vi "Counter_PulseWidthMeasurement.vi"() -> ()   [LabVIEW 2020]
uses:
  <userlib>/DAQNavi Polymorphic VI/create/DAQNavi Create Channel(CI-PulseWidth).vi
  <userlib>/DAQNavi Polymorphic VI/read/DAQNavi Read (Counter Pulse Width 1Chan 1Samp).vi
panel:
  in  "physical channels":string="PCI-1780,BID#0/cntr0" caption="property value"
  out "data":cluster{"high period":dbl, "low period":dbl}
  in  "stop":bool
  # "Please modify physical channels in Channel Parameters through DAQNavi Property Assistant VI  in block diagram."
  # "Channel Parameters"
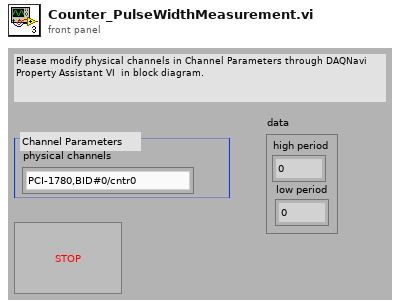
[diagram p1: front panel]
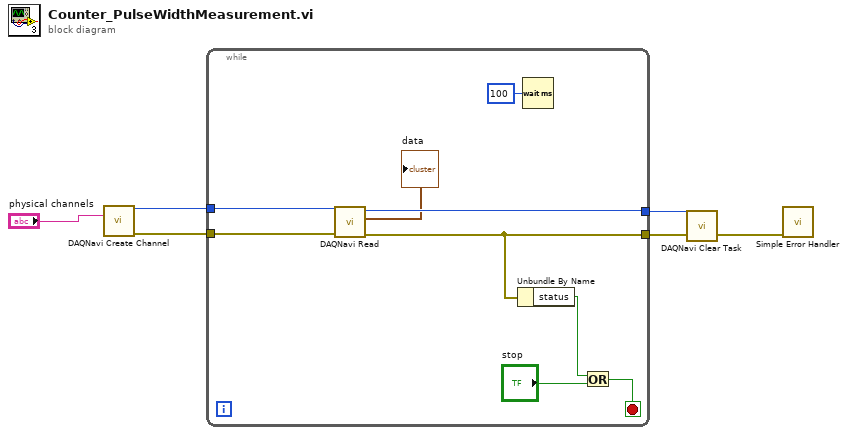
[diagram p0: block diagram]
diagram:
  n1 = call-poly <userlib>:"DAQNavi Create Channel.vi"("physical channels"="physical channels") -> ("task out"=w5:i32, "error out"=w4:errorcluster)  [unwired: 4 in, 9 out]
  n2 = while {
    tunnel: w5 -> [w15]
    tunnel: w4 -> [w14]
    tunnel: [w13] -> w3
    tunnel: [w11] -> w2
    stop <- w9 stop-if-true
    n3 = call-poly <userlib>:"DAQNavi Read.vi"("error in (no error)"=w14, "task in"=w15) -> ("error out"=w11:errorcluster, "data"=→"data":cluster{"high period":dbl, "low period":dbl}, "task out"=w13:i32)  [unwired: 2 in, 5 out]
    n4 = Unbundle By Name(w11) -> ("status"=w10:bool)
    n5 = Wait (ms)(milliseconds to wait=u32 100) -> ()  [unwired: 1 out]
    n6 = Or(x=w10, y="stop") -> (x .or. y?=w9:bool)
  }
  n7 = call <userlib>:"DAQNavi Clear Task.vi"("error in (no error)"=w2, "task in"=w3) -> ("error out"=w6:errorcluster)  [unwired: 1 out]
  n8 = call <vilib>:"Simple Error Handler.vi"("error in (no error)"=w6) -> ()  [unwired: 2 in, 7 out]
